vi "LBCB Position Popup.vi"(8 "error in (no error)":errorcluster, 11 "LBCB Number":T2) -> (0 "error out":errorcluster)   [LabVIEW 2009]
uses:
  lib/Data Access Objects/Metadata/LBCB Position.ctl
  lib/Data Access Objects/Metadata/LBCB Number.ctl
  Update Actions.ctl
  lib/Data Access Objects/Application/Number Of LBCBs.ctl
  lib/Data Access Objects/Metadata/Persistant DAO Actions.ctl
panel:
  in  "L2 Default LBCB Position":T1={"Motion Center"=[0.0, 0.0, 0.0], "Transformation Matrix"=[[1.0, 0.0, 0.0, 0.0, 0.0, 0.0], [0.0, 1.0, 0.0, 0.0, 0.0, 0.0], [0.0, 0.0, 1.0, 0.0, 0.0, 0.0], [0.0, 0.0, 0.0, 1.0, 0.0, 0.0], [0.0, 0.0, 0.0, 0.0, 1.0, 0.0], [0.0, 0.0, 0.0, 0.0, 0.0, 1.0]]} caption="Control Setting"
  in  "L1 Default LBCB Position":T1={"Motion Center"=[0.0, 0.0, 0.0], "Transformation Matrix"=[[1.0, 0.0, 0.0, 0.0, 0.0, 0.0], [0.0, 1.0, 0.0, 0.0, 0.0, 0.0], [0.0, 0.0, 1.0, 0.0, 0.0, 0.0], [0.0, 0.0, 0.0, 1.0, 0.0, 0.0], [0.0, 0.0, 0.0, 0.0, 1.0, 0.0], [0.0, 0.0, 0.0, 0.0, 0.0, 1.0]]} caption="Control Setting"
  in  "Cancel":bool
  in  "Ok":bool
  in  "LBCB Position":T1={"Motion Center"=[0.0, 0.0, 0.0], "Transformation Matrix"=[[1.0, 0.0, 0.0, 0.0, 0.0, 0.0], [0.0, 1.0, 0.0, 0.0, 0.0, 0.0], [0.0, 0.0, 1.0, 0.0, 0.0, 0.0], [0.0, 0.0, 0.0, 1.0, 0.0, 0.0], [0.0, 0.0, 0.0, 0.0, 1.0, 0.0], [0.0, 0.0, 0.0, 0.0, 0.0, 1.0]]} caption="Control Setting"
  # "(inch)"
  # "X"
  # "(inch)"
  # "Y"
  # "(inch)"
  # "Z"
  # "Xglobal = T*Xlocal"
  # "(inch)"
  # "X"
  # "(inch)"
  # "Y"
  # "(inch)"
  # "Z"
  # "Xglobal = T*Xlocal"
  # "Y"
  # "(inch)"
  # "XLBCB CMD = T-1*XLBCB OM"
  # "Z"
  # "(inch)"
  # "XOM DISP = T*XLBCB DISP"
  # "(inch)"
  # "Dx"
  # "Dy"
  # "Dz"
  # "Rx"
  # "Ry"
  # "Rz"
  # "Dx"
  # "Dy"
  # "Dz"
  # "Rx"
  # "Ry"
  # "Rz"
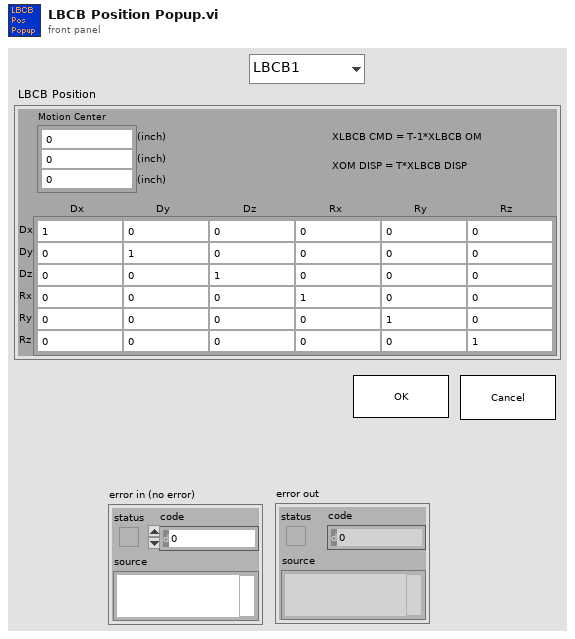
[diagram p1: front panel]
types:
  T1 = typedef "LBCB Position.ctl" = cluster{"Motion Center":dbl[], "Transformation Matrix":dbl[][]}
  T2 = typedef "LBCB Number.ctl" = enum16{"LBCB1", "LBCB2"}
  T3 = typedef "Update Actions.ctl" = enum16{"Update", "Exit"}
  T4 = enum8{"Enabled", "Disabled", "Disabled and Grayed Out"}
  T5 = typedef "Number Of LBCBs.ctl" = enum16{"1", "2"}
  T6 = typedef "Persistant DAO Actions.ctl" = enum16{"Init", "Get", "Set", "Load", "Save"}
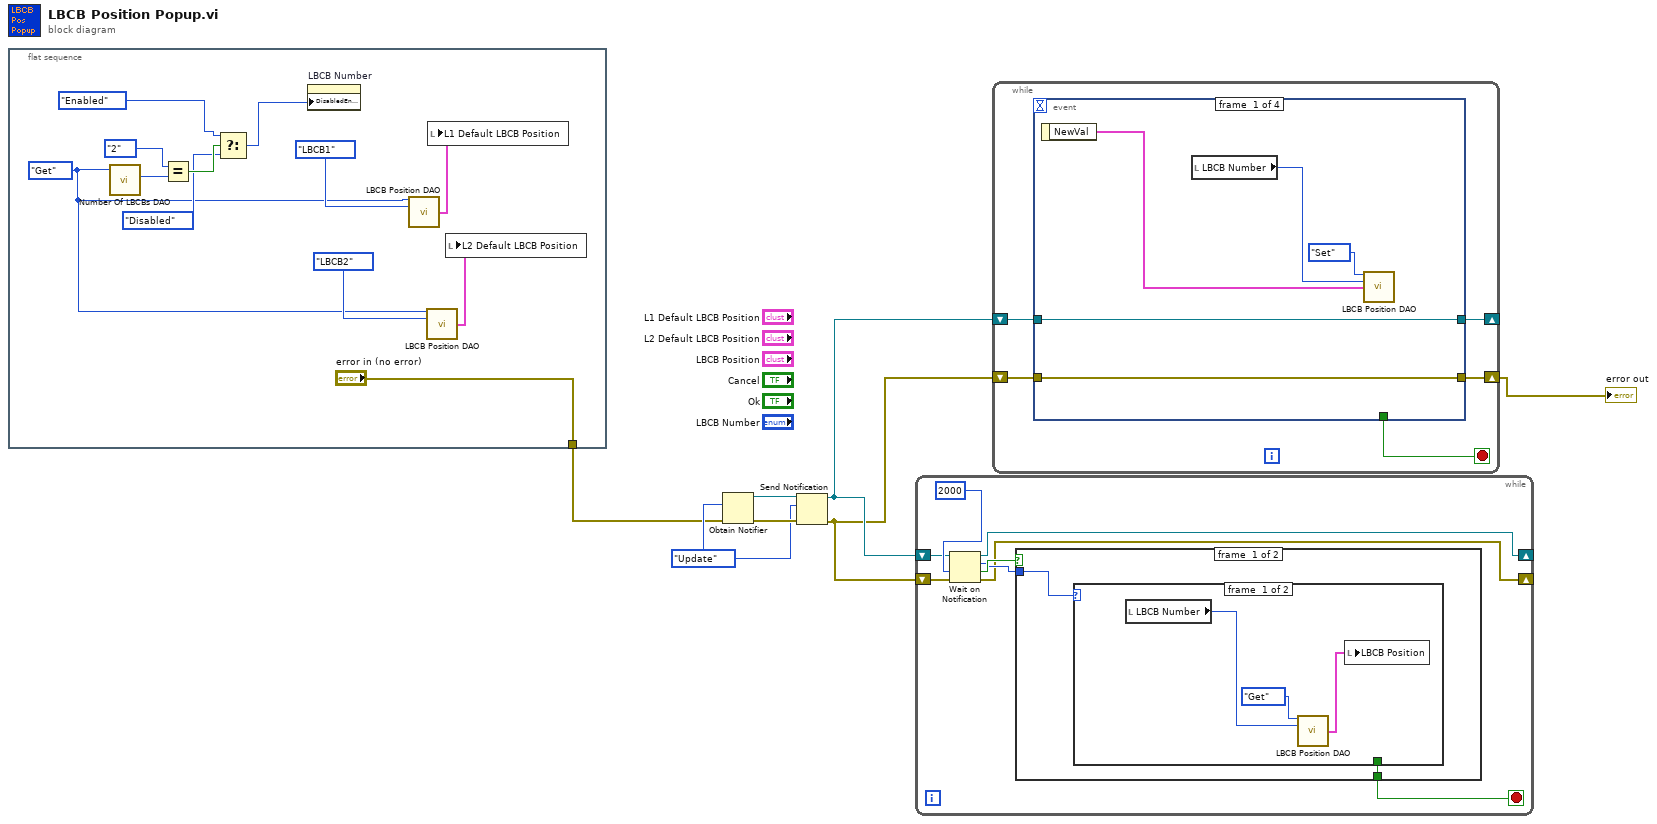
[diagram p0: block diagram]
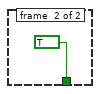
[diagram p2: hidden frame]
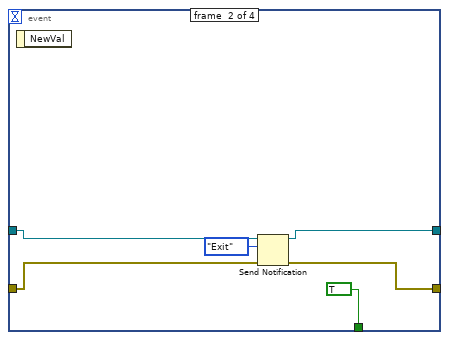
[diagram p4: hidden frame]
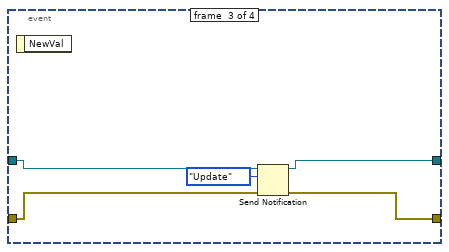
[diagram p5: hidden frame]
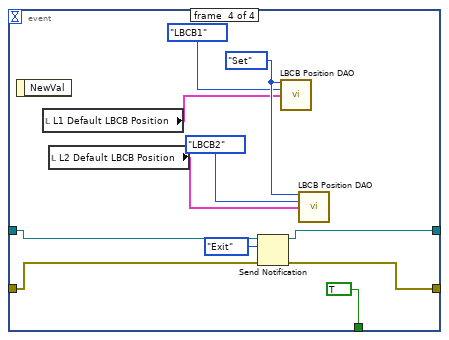
[diagram p6: hidden frame]
diagram:
  w5 = Update_Actions."Update" ("Update Actions")
  n1 = flat-sequence {
    tunnel: ["error in (no error)"] -> w4
    frame #0 {
      w9 = Persistant_DAO_Actions."Get" ("LBCB Settings Actions")
      n2 = call "Number Of LBCBs DAO.vi"("Actions"=w9) -> ("Number of\nLBCBs Out"=w14:T5)  [unwired: 7 in, 3 out]
      n3 = Equal?(x=Number_Of_LBCBs."2", y=w14) -> (x = y?=w12:bool)
      n4 = Select(t=T4."Enabled" ("Disabled"), s=w12, f=T4."Disabled") -> (s? t:f=w8:T4)
      n5 = property on="LBCB Number" class="Enum (strict)"("DisabledEnum"=w8) -> ()  [unwired: 2 in, 2 out]
      n6 = call "LBCB Position DAO.vi"("LBCB Settings Actions"=w9, "LBCB Number"=LBCB_Number."LBCB1") -> ("LBCB Position Output"=w19:T1)  [unwired: 3 in, 10 out]
      n7 = call "LBCB Position DAO.vi"("LBCB Settings Actions"=w9, "LBCB Number"=LBCB_Number."LBCB2") -> ("LBCB Position Output"=w17:T1)  [unwired: 3 in, 10 out]
      n8 = local write "L1 Default LBCB Position"(w19) -> ()
      n9 = local write "L2 Default LBCB Position"(w17) -> ()
    }
  }
  n10 = Obtain Notifier(notification data type=w5, error in (no error)=w4) -> (notifier out=w6:refnum<notifier>, error out=w7:errorcluster)  [unwired: 1 in, 2 out]
  n11 = Send Notification(notification=w5, notifier=w6, error in (no error)=w7) -> (notifier out=w3:refnum<notifier>, error out=w2:errorcluster)
  n12 = while {
    shift-right: [w21] -> _
    shift-left: w2 -> [w26]
    shift-right: [w22] -> _
    shift-left: w3 -> [w25]
    stop <- w20 stop-if-true
    n13 = Wait on Notification(notifier=w25, timeout in ms (-1)=2000, error in (no error)=w26) -> (notifier out=w22:refnum<notifier>, notification=w23:T3, timed out?=w24:bool, error out=w21:errorcluster)  [unwired: 1 out]
    n14 = case shown="False" w24 {
      tunnel: w23 -> [w29 _]
      tunnel: [w28 _] -> w20
      frame #0 {
        n15 = case shown="\"Exit\"" w29 {
          tunnel: [_ TRUE] -> w28
          frame #0 {
            n16 = local read "LBCB Number"() -> (w30:T2)
            n17 = call "LBCB Position DAO.vi"("LBCB Settings Actions"=Persistant_DAO_Actions."Get", "LBCB Number"=w30) -> ("LBCB Position Output"=w31:T1)  [unwired: 3 in, 10 out]
            n18 = local write "LBCB Position"(w31) -> ()
          }
          frame #1 {
          }
        }
      }
      frame #1 {
      }
    }
  }
  n19 = while {
    shift-right: [w35] -> _
    shift-left: w3 -> [w37]
    shift-right: [w34] -> w1
    shift-left: w2 -> [w36]
    stop <- w38 stop-if-true
    n20 = event shown="[3] \"Cancel\": Value Change" {
      selector: _ -> [_ _ _ _]
      dyn-events: _ -> [_ _ _ _]
      timeout: _ -> [_ _ _ _]
      tunnel: [_ TRUE _ TRUE] -> w38
      tunnel: w37 -> [w40 w48 w54 w64]
      tunnel: w36 -> [w39 w47 w53 w63]
      tunnel: [w40 w46 w52 w62] -> w35
      tunnel: [w39 w45 w51 w61] -> w34
      event #0 {
        n21 = event-data() -> ("NewVal"=w41:T1)  [unwired: 1 out]
        n22 = local read "LBCB Number"() -> (w43:T2)
        n23 = call "LBCB Position DAO.vi"("LBCB Settings Actions"=Persistant_DAO_Actions."Set", "LBCB Number"=w43, "LBCB Position In"=w41) -> ()  [unwired: 2 in, 11 out]
      }
      event #1 {
        n24 = event-data() -> ()  [unwired: 2 out]
        n25 = Send Notification(notification=Update_Actions."Exit", notifier=w48, error in (no error)=w47) -> (notifier out=w46:refnum<notifier>, error out=w45:errorcluster)
      }
      event #2 {
        n26 = event-data() -> ()  [unwired: 2 out]
        n27 = Send Notification(notification=Update_Actions."Update", notifier=w54, error in (no error)=w53) -> (notifier out=w52:refnum<notifier>, error out=w51:errorcluster)
      }
      event #3 {
        w59 = Persistant_DAO_Actions."Set" ("LBCB Settings Actions")
        n28 = event-data() -> ()  [unwired: 2 out]
        n29 = local read "L1 Default LBCB Position"() -> (w56:T1)
        n30 = local read "L2 Default LBCB Position"() -> (w55:T1)
        n31 = Send Notification(notification=Update_Actions."Exit", notifier=w64, error in (no error)=w63) -> (notifier out=w62:refnum<notifier>, error out=w61:errorcluster)
        n32 = call "LBCB Position DAO.vi"("LBCB Settings Actions"=w59, "LBCB Number"=LBCB_Number."LBCB1", "LBCB Position In"=w56) -> ()  [unwired: 2 in, 11 out]
        n33 = call "LBCB Position DAO.vi"("LBCB Settings Actions"=w59, "LBCB Number"=LBCB_Number."LBCB2", "LBCB Position In"=w55) -> ()  [unwired: 2 in, 11 out]
      }
    }
  }
  "error out" <- w1
